vi "AAA Generics, Catalog.vi"   [LabVIEW 2010]
panel:
  # "Generics\nCatalog"
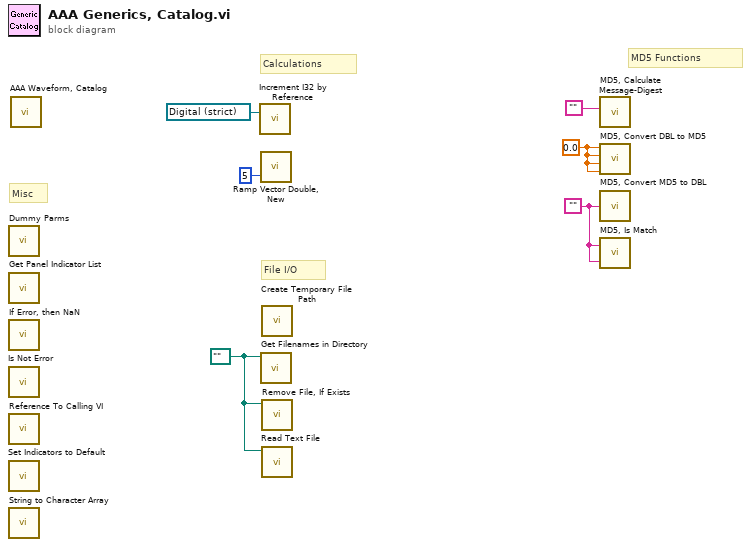
[diagram p0: block diagram]
diagram:
  w1 = path "" ("directory path")
  w6 = 0.0 ("MD5[0]")
  w4 = ""
  # "MD5 Functions"
  # "Misc"
  # "File I/O"
  # "Calculations"
  n1 = call "Dummy Parms.vi"() -> ()  [unwired: 6 in, 6 out]
  n2 = call "Get Panel Indicator List.vi"() -> ()  [unwired: 5 in, 3 out]
  n3 = call "If Error, then NaN.vi"() -> ()  [unwired: 6 in, 4 out]
  n4 = call "Is Not Error.vi"() -> ()  [unwired: 6 in, 3 out]
  n5 = call "Reference To Calling VI.vi"() -> ()  [unwired: 3 in, 2 out]
  n6 = call "Set Indicators to Default.vi"() -> ()  [unwired: 7 in, 1 out]
  n7 = call "String to Character Array.vi"() -> ()  [unwired: 1 in, 1 out]
  n8 = call "AAA Waveform, Catalog.vi"() -> ()  [unwired: 12 in]
  n9 = call "Increment I32 by Reference.vi"("dignum refnum"=refnum<vi> refnum) -> ()  [unwired: 7 in, 3 out]
  n10 = call "Ramp Vector Double, New.vi"("nelem"=5) -> ()  [unwired: 2 in, 1 out]
  n11 = call "Get Filenames in Directory.vi"("directory path"=w1) -> ()  [unwired: 9 in, 2 out]
  n12 = call "Create Temporary File Path.vi"() -> ()  [unwired: 6 in, 2 out]
  n13 = call "Remove File, If Exists.vi"("filepath"=w1) -> ()  [unwired: 5 in, 2 out]
  n14 = call "Read Text File.vi"("filepath"=w1) -> ()  [unwired: 8 in, 3 out]
  n15 = call "MD5, Calculate Message-Digest.vi"("data"="") -> ()  [unwired: 3 in, 1 out]
  n16 = call "MD5, Convert DBL to MD5.vi"("MD5[0]"=w6, "MD5[1]"=w6, "MD5[2]"=w6, "MD5[3]"=w6) -> ()  [unwired: 2 out]
  n17 = call "MD5, Convert MD5 to DBL.vi"("MD5"=w4) -> ()  [unwired: 5 out]
  n18 = call "MD5, Is Match.vi"("MD5(b)"=w4, "MD5(a)"=w4) -> ()  [unwired: 6 out]
